vi "Simple Get.vi"   [LabVIEW 2017, in "NI_WebDAV.lvlib"]
doc: "Returns a file or multiple files or the raw binary contents of a file or multiple files from a remote WebDAV server or target. You must manually select the polymorphic instance you want to use."
uses:
  <vilib>/WebDAVClient/NI_WebDAV.lvlib
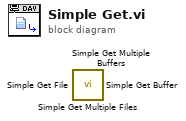
[diagram p0: block diagram]
diagram:
  n1 = call <vilib>:"Simple Get Multiple Files.vi"() -> ()  [unwired: 15 in, 1 out]
  n2 = call <vilib>:"Simple Get Multiple Buffers.vi"() -> ()  [unwired: 14 in, 2 out]
  n3 = call <vilib>:"Simple Get File.vi"() -> ()  [unwired: 14 in, 2 out]
  n4 = call <vilib>:"Simple Get Buffer.vi"() -> ()  [unwired: 14 in, 2 out]
